vi "Actor Core.vi"(8 "error in":errorcluster, 11 "Table in":refnum<class "Table.lvclass">) -> (0 "error out":errorcluster, 3 "Table out":refnum<class "Actor.lvclass">)   [LabVIEW 2023, in "Table.lvlib" / "Table.lvclass"]
uses:
  Table.lvclass
  C:/Program Files (x86)/National Instruments/LabVIEW 2023/vi.lib/ActorFramework/Actor/Actor.lvclass
  <vilib>/ActorFramework/Actor/Actor.lvclass
  Table.lvclass/Table.ctl
  Philosopher/Philosopher/Philosopher.lvclass
  Fork.ctl
  Hungry.ctl
  <vilib>/ActorFramework/Actor/Actor.lvclass/Actor.ctl
  <vilib>/ActorFramework/Message Enqueuer/Message Enqueuer.lvclass/Message Enqueuer.ctl
  d5f59e19-9d9d-4156-8b99-cb3ddaf3303d.vi
  <vilib>/ActorFramework/Message Enqueuer/Enqueue.vi
  <vilib>/ActorFramework/Message Enqueuer/Init from Existing Queue.vi
  <vilib>/ActorFramework/Stop Msg/Stop Msg.lvclass
  C:/Program Files (x86)/National Instruments/LabVIEW 2023/vi.lib/ActorFramework/Message/Message.lvclass
  Philosopher/Philosopher Messages/Timeout Hungry/Timeout Eating Msg.lvclass
  <vilib>/Utility/LVClass/Get LV Class Name.vi
  <resource>/AFDebug/Generate Trace for Message.vi
  <vilib>/ActorFramework/Message Priority Queue/Priority Enqueue.vi
  <vilib>/ActorFramework/Message Enqueuer/Message Enqueuer.lvclass
panel:
  in  "stop signal":bool
  in  "The End":bool
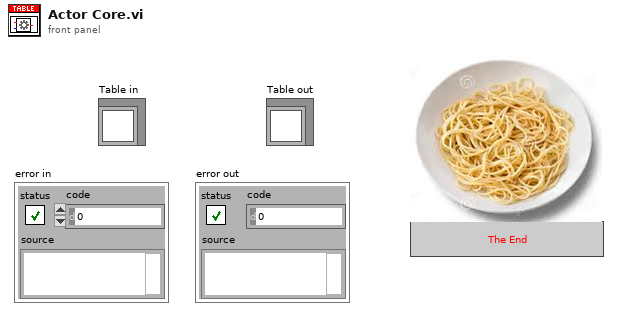
[diagram p1: front panel]
types:
  T1 = typedef "Table.lvlib/Table.lvclass/Hungry.ctl" = enum16{"NO", "YES"}
  T2 = typedef "Table.lvlib/Table.lvclass/Fork.ctl" = enum16{"FREE", "IN USE"}
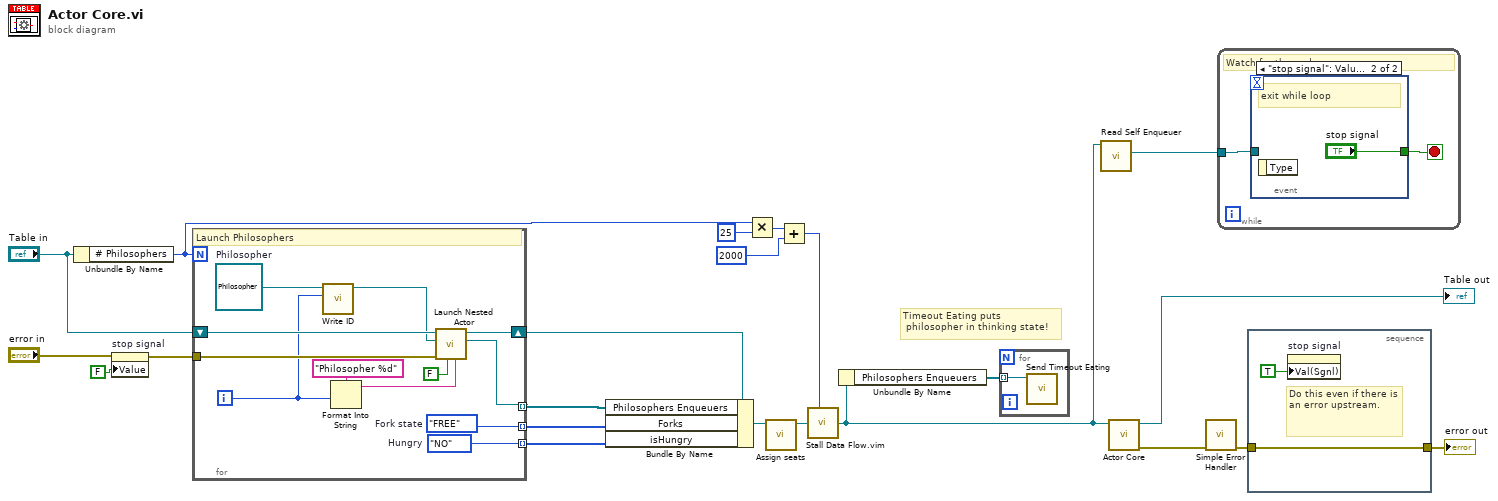
[diagram p0: block diagram]
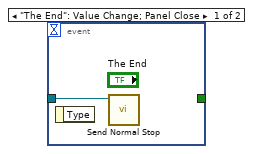
[diagram p2: hidden frame]
diagram:
  # "Timeout Eating puts\n philosopher in thinking state!"
  n1 = Unbundle By Name("Table in") -> ("# Philosophers"=w5:i32)
  n2 = property on="stop signal" class="Bool (strict)"(error in="error in", "Value"=FALSE ("stop")) -> (error out=w14:errorcluster)  [unwired: 1 in, 1 out]
  n3 = for {
    N: w5 -> [_]
    tunnel: w14 -> [w33]
    shift-right: [w31] -> w12
    shift-left: "Table in" -> [w32]
    tunnel: [w30] -> w17 mode=indexing
    tunnel: [w29] -> w16 mode=indexing
    tunnel: [w28] -> w11 mode=indexing
    i -> [w24]
    w29 = Hungry."NO"  # Hungry
    w30 = Fork."FREE"  # Fork state
    w25 = refnum<class "Philosopher.lvclass"> refnum  # Philosopher
    # "Launch Philosophers"
    n4 = call-dynamic "Write ID.vi"("ID"=w24, "Philosopher in"=w25) -> ("Philosopher out"=w23:refnum<class "Philosopher.lvclass">)  [unwired: 8 in, 1 out]
    n5 = Format Into String(format string="Philosopher %d", w24) -> (resulting string=w26:string)  [unwired: 2 in, 1 out]
    n6 = call <vilib>:"Launch Nested Actor.vi"("Debug Alias"=w26, "Open Actor Core front panel? (F)"=FALSE, "error in (no error)"=w33, "Nested Actor"=w23, "Caller Actor in"=w32) -> ("Nested Actor's Enqueuer"=w28:refnum<class "Message Enqueuer.lvclass">, "Caller Actor out"=w31:refnum<class "Table.lvclass">)  [unwired: 4 in, 1 out]
  }
  n7 = Bundle By Name(cluster=w12, "Philosophers Enqueuers"=w11, "Forks"=w17, "isHungry"=w16) -> (w10:refnum<class "Table.lvclass">)
  n8 = Multiply(x=w5, y=25) -> (x*y=w3:i32)
  n9 = call-dynamic "Assign seats.vi"("Table in"=w10) -> ("Table out"=w7:refnum<class "Table.lvclass">)  [unwired: 9 in, 1 out]
  n10 = Add(x=w3, y=u32 2000 ("milliseconds to wait")) -> (x+y=w1:u32)
  n11 = call "Stall Data Flow.vim"("value in"=w7, "milliseconds to wait"=w1) -> ("value out"=w6:refnum<class "Table.lvclass">)  [unwired: 1 out]
  n12 = Unbundle By Name(w6) -> ("Philosophers Enqueuers"=w8:refnum<class "Message Enqueuer.lvclass">[])
  n13 = for {
    tunnel: w8 -> [w35] mode=indexing
    n14 = call "Send Timeout Eating.vi"("Message Enqueuer"=w35) -> ()  [unwired: 9 in, 2 out]
  }
  n15 = call <vilib>:"Read Self Enqueuer.vi"("Actor"=w6) -> ("Self Enqueuer"=w19:refnum<class "Message Enqueuer.lvclass">)  [unwired: 10 in]
  n16 = call-parent "Actor Core.vi"("Actor in"=w6) -> ("error out"=w21:errorcluster, "Actor out"=→"Table out":refnum<class "Actor.lvclass">)  [unwired: 9 in]
  n17 = call <vilib>:"Simple Error Handler.vi"("error in (no error)"=w21) -> ("error out"=w18:errorcluster)  [unwired: 4 in, 4 out]
  n18 = while {
    tunnel: w19 -> [w37]
    stop <- w36 stop-if-true
    # "Watch for the end"
    n19 = event shown="[1] \"stop signal\": Value Change" {
      selector: _ -> [_ _]
      dyn-events: _ -> [_ _]
      timeout: _ -> [_ _]
      tunnel: w37 -> [w38 _]
      tunnel: [_ "stop signal"] -> w36
      event "The End": Value Change; Panel Close {
        n20 = event-data() -> ()  [unwired: 1 in, 1 out]
        n21 = call <vilib>:"Send Normal Stop.vi"("Message Enqueuer"=w38) -> ()  [unwired: 10 in, 1 out]
      }
      event "stop signal": Value Change {
        # "exit while loop"
        n22 = event-data() -> ()  [unwired: 1 in, 1 out]
      }
    }
  }
  n23 = stacked-sequence {
    tunnel: [w40] -> w13
    tunnel: w18 -> [w40]
    frame #0 {
      # "Do this even if there is an error upstream."
      n24 = property on="stop signal" class="Bool (strict)"("Val(Sgnl)"=TRUE ("stop")) -> ()  [unwired: 2 in, 2 out]
    }
  }
  "error out" <- w13
